vi "GetFileStringTiff.vi"(7 "Color Palette":T2[](array[typedef]), 8 "error in":errorcluster, 9 "Base64 Encoded":bool, 10 "TIFF Options":T1={"Rows Per Strip"=0.0, "Photometric"=1, "Compression Type"=0} {"Compression Type" items=["None", "JPEG", "Run Length Encoded", "Zip"]; "Photometric" items=["WhiteIsZero", "BlackIsZero"]}, 11 "Image Reference In":T3) -> (0 "error out":errorcluster, 2 "FileString":string, 3 "Image Reference Out":T3)   [LabVIEW 2024, in "OpenLvVision_Image.lvlib" / "File.lvlib"]
doc: "Returns the entire image content encoded as a string representing an image file, suitable for saving or transferring over the network."
uses:
  File.lvlib
  Management/TypeDef/Image.ctl
  TypeDef/ColorPaletteValue.ctl
  TypeDef/TiffOptions.ctl
  Management/Management.lvlib
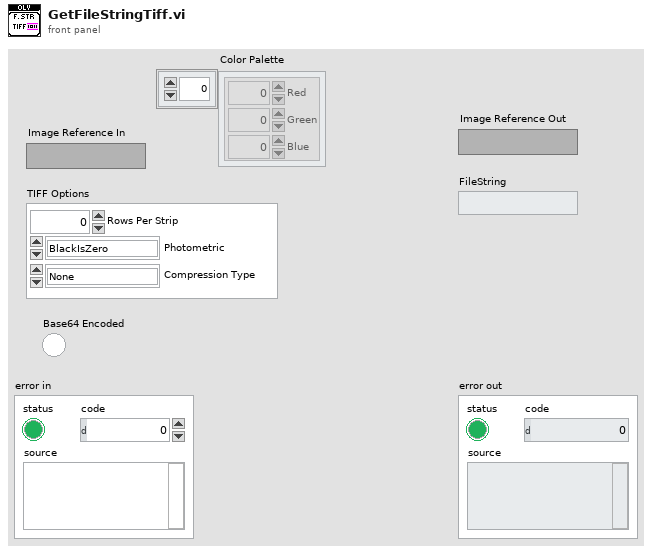
[diagram p1: front panel]
types:
  T1 = typedef "OpenLvVision_Image.lvlib/File.lvlib/TiffOptions.ctl" = cluster{"Rows Per Strip":dbl, "Photometric":i32, "Compression Type":i32}
  T2 = typedef "OpenLvVision_Image.lvlib/File.lvlib/ColorPaletteValue.ctl" = cluster{"Red":u8, "Green":u8, "Blue":u8}
  T3 = typedef "OpenLvVision_Image.lvlib/Management.lvlib/Image.ctl" = refnum<image>
  T4 = typedef "IMAQ Image.ctl" = refnum<image>
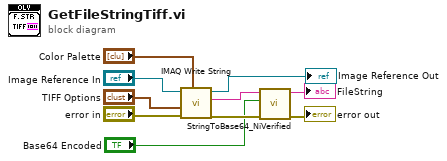
[diagram p0: block diagram]
diagram:
  n1 = call-poly "IMAQ Write String"("Color Palette"="Color Palette", "error in (no error)"="error in", "TIFF Options"="TIFF Options", "Image"="Image Reference In") -> ("error out"=w5:errorcluster, "FileString"=w2:string, "Image Out (duplicate)"=→"Image Reference Out":T4)  [unwired: 5 in]
  n2 = call "StringToBase64_NiVerified.vi"("error in"=w5, "Encode"="Base64 Encoded", "RawString"=w2) -> ("error out"=→"error out":errorcluster, "EncodedString"=→"FileString":string)  [unwired: 7 in]
